vi "Sub Initialize.vi"(8 "error in (no error)":errorcluster, 11 "Measure Object in":refnum<class "Process Object.lvclass">) -> (0 "error out":errorcluster, 2 "Initialize Result":refnum<class "Acquired Result.lvclass">, 3 "Measure Object out":refnum<class "Process Object.lvclass">)   [LabVIEW 2016, in "Process Object.lvclass"]
uses:
  Process Object.lvclass
  C:/Program Files (x86)/National Instruments/LabVIEW 2016/vi.lib/ActorFramework/Actor/Actor.lvclass
  NHMFL_Core/Libraries/Instruments/Results/Acquired Result/Acquired Result.lvclass
  Process Object.lvclass/Process Object.ctl
  <vilib>/ActorFramework/Actor/Actor.lvclass/Actor.ctl
  <vilib>/ActorFramework/Message Enqueuer/Message Enqueuer.lvclass/Message Enqueuer.ctl
  Template Module Messages/Subscribe Request Msg/Subscribe Request Msg.lvclass/Subscribe Request Msg.ctl
  Read Broadcaster name.vi
  Write Result ready.vi
  <vilib>/ActorFramework/Message Enqueuer/Init from Existing Queue.vi
  <vilib>/ActorFramework/Message Enqueuer/Enqueue.vi
  Template Module Messages/Subscribe Request Msg/Subscribe Request Msg.lvclass
  C:/Program Files (x86)/National Instruments/LabVIEW 2016/vi.lib/ActorFramework/Message/Message.lvclass
  <vilib>/ActorFramework/Message Priority Queue/Priority Enqueue.vi
  Worker/Worker.lvclass
  <vilib>/ActorFramework/Message Enqueuer/Message Enqueuer.lvclass
  <vilib>/ActorFramework/Actor/Actor.lvclass
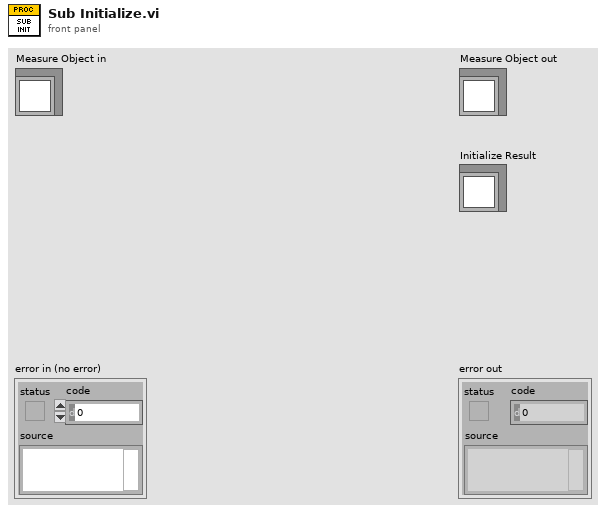
[diagram p1: front panel]
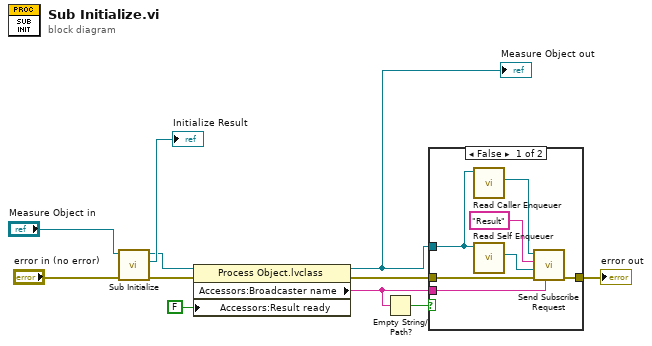
[diagram p0: block diagram]
diagram:
  n1 = call-parent "Sub Initialize.vi"("error in (no error)"="error in (no error)", "Measure Object in"="Measure Object in") -> ("error out"=w7:errorcluster, "Initialize Result"=→"Initialize Result":refnum<class "Acquired Result.lvclass">, "Measure Object out"=w5:refnum<class "Process Object.lvclass">)  [unwired: 7 in]
  n2 = property class="Process Object.lvclass"(reference=w5, error in=w7, "Accessors:Result ready"=FALSE ("Result ready")) -> (reference out=w4:refnum<class "Process Object.lvclass">, error out=w9:errorcluster, "Accessors:Broadcaster name"=w2:string)
  "Measure Object out" <- w4
  n3 = Empty String/Path?(string/path=w2) -> (empty?=w1:bool)
  n4 = case shown="False" w1 {
    tunnel: w9 -> [w18 w19]
    tunnel: [w14 w19] -> w8
    tunnel: w2 -> [w13 _]
    tunnel: w4 -> [w12 _]
    frame False {
      n5 = call <vilib>:"Read Caller Enqueuer.vi"("Actor"=w12) -> ("Caller Enqueuer"=w16:refnum<class "Message Enqueuer.lvclass">)  [unwired: 10 in]
      n6 = call <vilib>:"Read Self Enqueuer.vi"("Actor"=w12) -> ("Self Enqueuer"=w17:refnum<class "Message Enqueuer.lvclass">)  [unwired: 10 in]
      n7 = call "Send Subscribe Request.vi"("Broadcaster"=w13, "error in (no error)"=w18, "Subscriber Enqueuer"=w17, "Topic"="Result", "Message Enqueuer"=w16) -> ("error out"=w14:errorcluster)  [unwired: 5 in, 1 out]
    }
    frame True {
    }
  }
  "error out" <- w8
